vi "setTestCaseInstanceName.vi"(10 "Test Case Instance Name (<Class Name>)":string, 11 "TestCase in":refnum<class "TestCase.lvclass">) -> (3 "TestCase out":refnum<class "TestCase.lvclass">)   [LabVIEW 2013, in "TestCase.lvclass"]
doc: "Sets the name for this instance of the test case. This is the name that will appear in the user interface."
uses:
  TestCase.lvclass
  TestCase.lvclass/TestCase.ctl
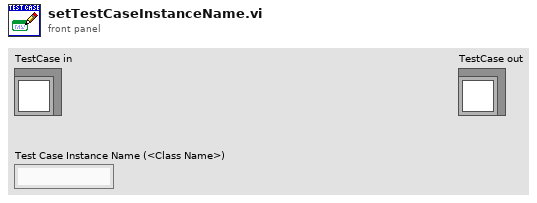
[diagram p1: front panel]
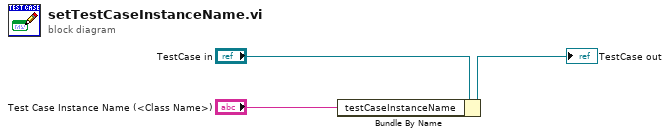
[diagram p0: block diagram]
diagram:
  n1 = Bundle By Name(cluster="TestCase in", "testCaseInstanceName"="Test Case Instance Name (<Class Name>)") -> (→"TestCase out":refnum<class "TestCase.lvclass">)
